vi "retrieve control values.vi"(8 "error in (no error)":errorcluster, 11 "User":string) -> (0 "error out":errorcluster)   [LabVIEW 2016]
panel:
  out "Variant":variant
  out "Name":string
  out "call chain":string[](array[string])
  out "value":T1(array[cluster])
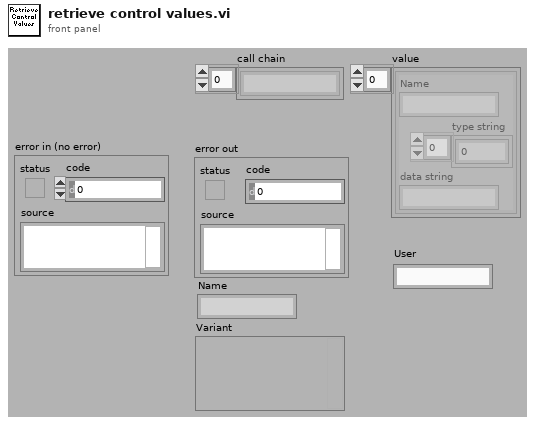
[diagram p1: front panel]
types:
  T1 = cluster{"Name":string, "type string":i16[], "data string":string}[]
  T2 = enum32{"invalid app kind", "Development System", "Run Time System", "Student Edition", "Embedded LabVIEW", "Evaluation", "Custom"}
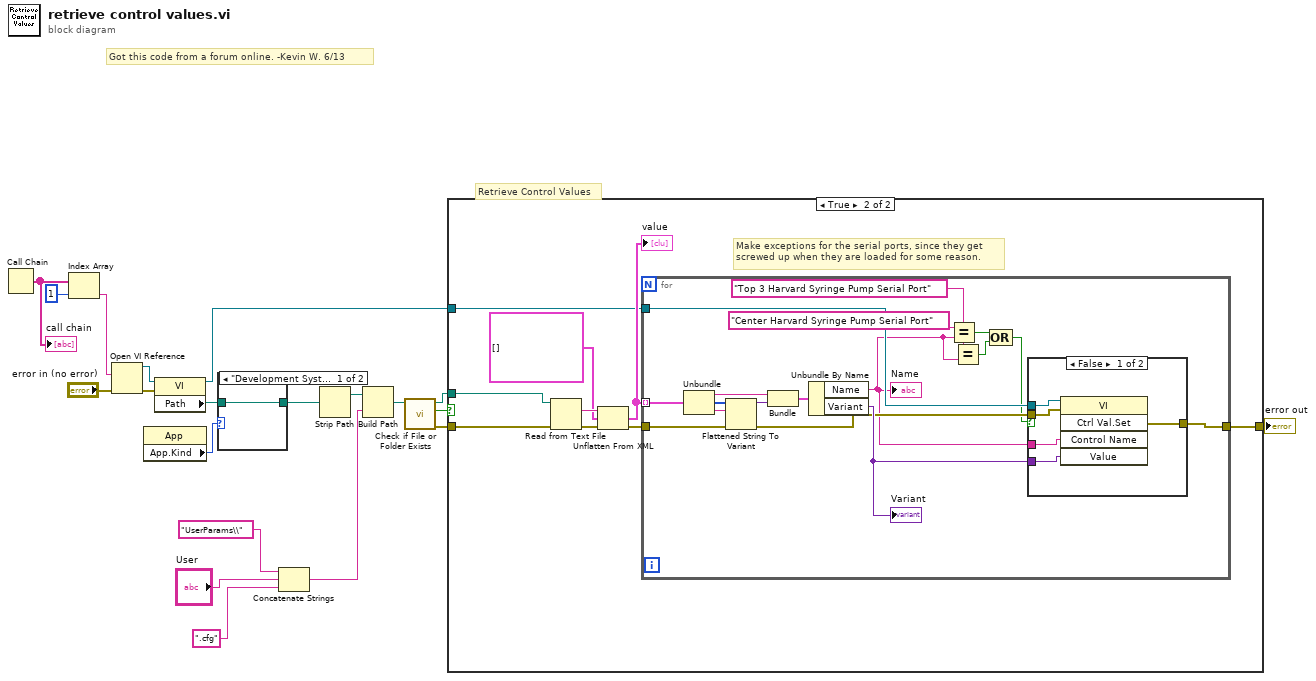
[diagram p0: block diagram]
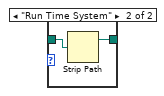
[diagram p2: hidden frame]
diagram:
  # "Got this code from a forum online. -Kevin W. 6/13"
  # "Retrieve Control Values"
  n1 = Call Chain() -> (call chain=w20:string[])
  "call chain" <- w20
  n2 = Index Array(array=w20, index=1) -> (element=w12:string)
  n3 = Open VI Reference(vi path=w12, error in (no error)="error in (no error)") -> (vi reference=w11:refnum<vi>, error out=w15:errorcluster)  [unwired: 4 in]
  n4 = property class="App"() -> ("App.Kind"=w7:T2)  [unwired: 2 in, 2 out]
  n5 = property class="VI"(reference=w11, error in=w15) -> (reference out=w5:refnum<vi>, "Path"=w8:path)  [unwired: 1 out]
  n6 = case shown="\"Development System\", Default" w7 {
    tunnel: w8 -> [w21 w23]
    tunnel: [w21 w22] -> w6
    frame "Development System", Default {
    }
    frame "Run Time System" {
      n7 = Strip Path(path=w23) -> (stripped path=w22:path)  [unwired: 1 out]
    }
  }
  n8 = Concatenate Strings("UserParams\\", "User", ".cfg") -> (w1:string)
  n9 = Strip Path(path=w6) -> (stripped path=w10:path)  [unwired: 1 out]
  n10 = Build Path(base path=w10, name or relative path=w1) -> (appended path=w9:path)
  n11 = call <vilib>:"Check if File or Folder Exists.vi"("path"=w9) -> ("error out"=w14:errorcluster, "file or folder exists?"=w17:bool, "dup path"=w18:path)  [unwired: 8 in]
  n12 = case shown="True" w17 {
    tunnel: w5 -> [_ w28]
    tunnel: w18 -> [_ w27]
    tunnel: w14 -> [w24 w26]
    tunnel: [w24 w25] -> w13
    frame False {
    }
    frame True {
      # "Make exceptions for the serial ports, since they get\nscrewed up when they are loaded for some reason."
      n13 = Read from Text File(file (use dialog)=w27, error in=w26) -> (text=w33:string, error out=w31:errorcluster)  [unwired: 4 out]
      n14 = Unflatten From XML(xml string=w33, type=T1 [], error in (no error)=w31) -> (value=w29:T1, error out=w32:errorcluster)
      "value" <- w29
      n15 = for {
        tunnel: w32 -> [w48]
        tunnel: [w49] -> w25
        tunnel: w29 -> [w45] mode=indexing
        tunnel: w28 -> [w41]
        n16 = Unbundle(w45) -> ("Name"=w46:string, "type string"=w44:i16[], "data string"=w43:string)
        n17 = Flattened String To Variant(4:w48, 6:w43, 7:w44) -> (0:w40:errorcluster, 3:w47:variant)
        n18 = Bundle("Name"=w46, "Variant"=w47) -> (w42:cluster{"Name":string, "Variant":variant})  [unwired: 1 out]
        n19 = Unbundle By Name(w42) -> ("Name"=w35:string, "Variant"=w50:variant)
        "Name" <- w35
        "Variant" <- w50
        n20 = Equal?(x="Center Harvard Syringe Pump Serial Port", y=w35) -> (x = y?=w39:bool)
        n21 = Equal?(x="Top 3 Harvard Syringe Pump Serial Port", y=w35) -> (x = y?=w34:bool)
        n22 = Compound Arithmetic op=OR(w39, w34) -> (w37:bool)
        n23 = case shown="False" w37 {
          tunnel: w50 -> [w55 _]
          tunnel: [w54 w56] -> w49
          tunnel: w35 -> [w53 _]
          tunnel: w41 -> [w52 _]
          tunnel: w40 -> [w51 w56]
          frame False {
            n24 = invoke class="VI" method="Ctrl Val.Set"(reference=w52, error in=w51, "Control Name"=w53, "Value"=w55) -> (error out=w54:errorcluster)  [unwired: 1 in, 4 out]
          }
          frame True {
          }
        }
      }
    }
  }
  "error out" <- w13
